vi "DSF.Transceiver.GE Reflective Memory.Get VISA Resource Name.vi"(11 "GE Reflective Memory in":refnum<class "DSF.Transceiver.GE Reflective Memory.lvclass">) -> (2 "VISA resource name":refnum<visa-resource-name>, 3 "GE Reflective Memory out":refnum<class "DSF.Transceiver.GE Reflective Memory.lvclass">)   [LabVIEW 2017, in "DSF.Transceiver.GE Reflective Memory.lvlib" / "DSF.Transceiver.GE Reflective Memory.lvclass"]
uses:
  DSF.Transceiver.GE Reflective Memory.lvclass
  DSF.Transceiver.GE Reflective Memory.lvclass/DSF.Transceiver.GE Reflective Memory.ctl
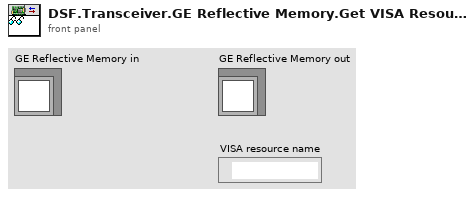
[diagram p1: front panel]
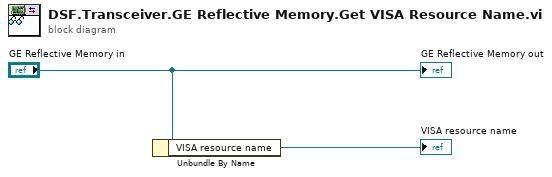
[diagram p0: block diagram]
diagram:
  n1 = Unbundle By Name("GE Reflective Memory in") -> ("VISA resource name"=→"VISA resource name":refnum<visa-resource-name>)
  "GE Reflective Memory out" <- "GE Reflective Memory in"
